vi "pport_turn_on_the_lights.vi"() -> ()   [LabVIEW 2011]
doc: "This example program uses the In Port.vi and Out Port.vi to continuously poll the parallel port's data, status, and control registers and update them when the user specifies. \n\nWhen using this VI it is necessary to first place the PC parallel port into standard mode (SPP) in the BIOS configuration and make note of the port's base address. This will require re-booting the PC. After this has been done, enter the parallel port base address into the Data Register (Base + 0) control on the IO Register Status tab and the VI is ready to be run.\n\nNOTE: In Port.vi and Out Port.vi, which this example uses, are not supported on Windows Vista and later."
uses:
  <vilib>/Utility/file.llb/Read From Spreadsheet File (I64).vi
  <vilib>/Platform/portaccess.llb/Out Port32.vi
  <vilib>/Platform/portaccess.llb/In Port32.vi
panel:
  out "Wait":i32
  out "Bit":i32
  out "Current trial":i32
  out "register data read":bool[](array[boolean])
  in  "address":i16=888 format="%.0x"
  out "Trials":i32=116
  in  "File path of timing delays from scan onset (ms)":path=path "C:/Work/Work/MC_LabVIEW_programs/Gregs_Piano/Practice Run Block_NEW.txt"
  # "Data Register (Base +0)"
  # "16      8                     1                  4         2\nLeft                                               Right\n\nNo lights = 0\nFor any other combination, just add up what you want\ne.g. 16 + 2 = 18 (Cue L and R outer)"
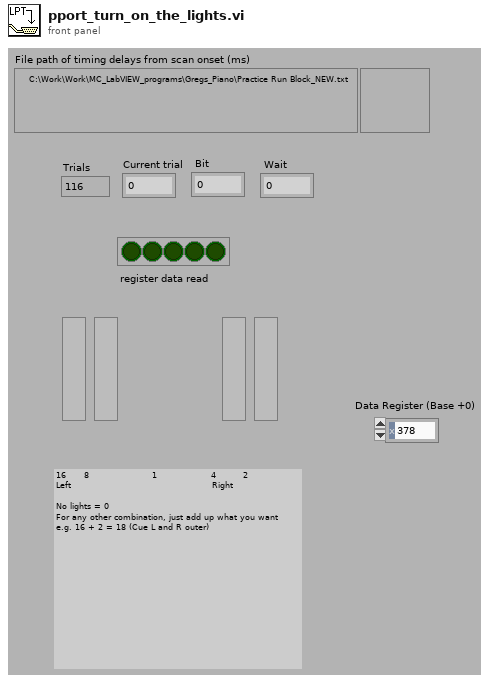
[diagram p1: front panel]
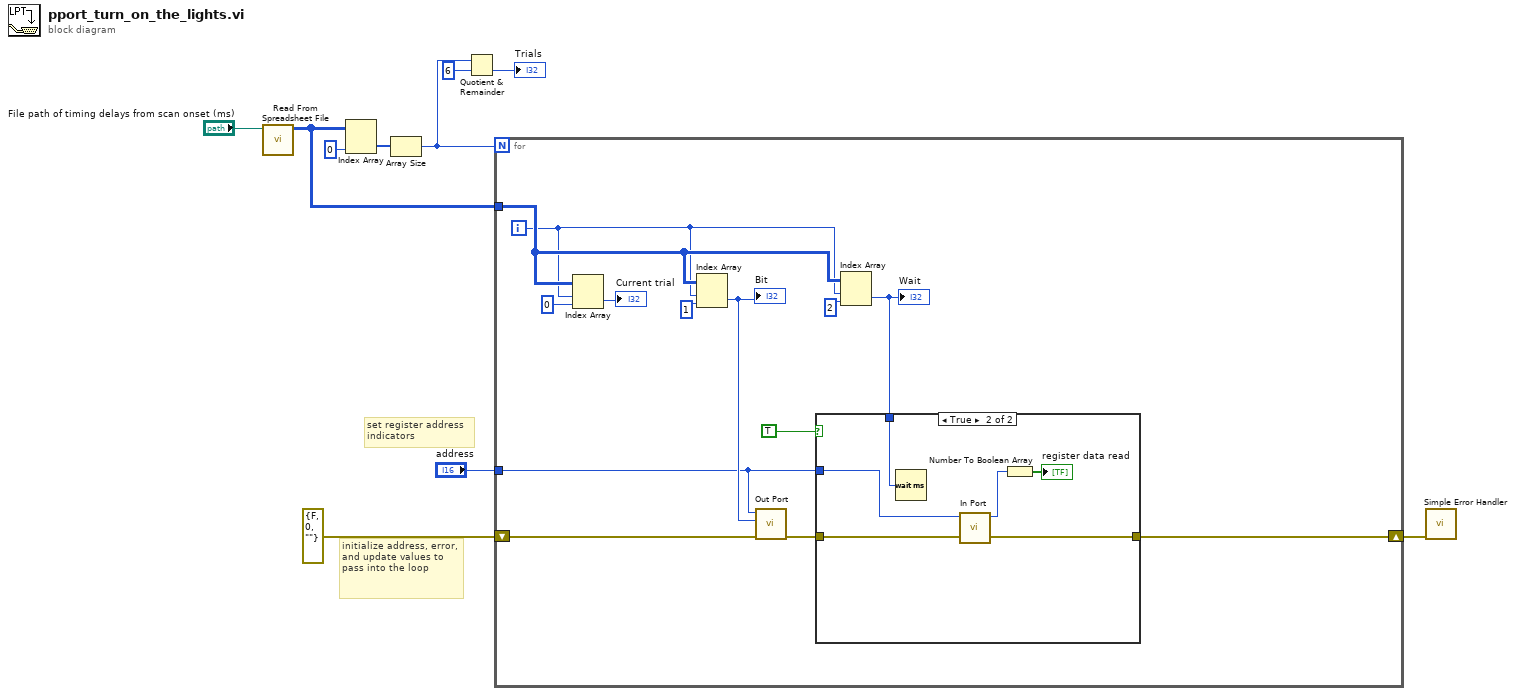
[diagram p0: block diagram]
diagram:
  # "initialize address, error,\nand update values to pass into the loop"
  # "set register address indicators"
  n1 = call-poly <vilib>:"Read From Spreadsheet File.vi"("file path (dialog if empty)"="File path of timing delays from scan onset (ms)") -> ("all rows"=w5:i64[][])  [unwired: 6 in, 4 out]
  n2 = Index Array(array=w5, index (col)=0 ("disabled index (col)")) -> (element=w8:i64[])  [unwired: 1 in]
  n3 = Array Size(array=w8) -> (size(s)=w3:i32)
  n4 = Quotient & Remainder(x=w3, y=6) -> (floor(x/y)=→"Trials":i32)  [unwired: 1 out]
  n5 = for {
    N: w3 -> [_]
    shift-right: [w13] -> w10
    shift-left: errorcluster {"status"=FALSE, "code"=0, "source"=""} ("error in") -> [w17]
    tunnel: w5 -> [w19]
    tunnel: "address" -> [w14]
    i -> [w11]
    n6 = Index Array(array=w19, index (row)=w11, index (col)=0 ("disabled index (col)")) -> (element=→"Current trial":i64)
    n7 = Index Array(array=w19, index (row)=w11, index (col)=1 ("disabled index (col)")) -> (element=w18:i64)
    "Bit" <- w18
    n8 = call-poly <vilib>:"Out Port.vi"("error in (no error)"=w17, "write value"=w18, "address"=w14) -> ("error out"=w15:errorcluster)  [unwired: 6 in]
    n9 = Index Array(array=w19, index (row)=w11, index (col)=2 ("disabled index (col)")) -> (element=w16:i64)
    "Wait" <- w16
    n10 = case shown="True" TRUE {
      tunnel: w16 -> [_ w29]
      tunnel: w15 -> [w24 w28]
      tunnel: w14 -> [_ w27]
      tunnel: [w24 w25] -> w13
      frame False {
      }
      frame True {
        n11 = Wait (ms)(milliseconds to wait=w29) -> ()  [unwired: 1 out]
        n12 = call-poly <vilib>:"In Port.vi"("error in (no error)"=w28, "address"=w27) -> ("error out"=w25:errorcluster, "data read"=w26:i32)  [unwired: 6 in]
        n13 = Number To Boolean Array(number=w26) -> (Boolean array=→"register data read":bool[])
      }
    }
  }
  n14 = call <vilib>:"Simple Error Handler.vi"("error in (no error)"=w10) -> ()  [unwired: 4 in, 5 out]
